vi "Set Last Temperatures.vi"(6 "Read Channel Ident":string, 8 "error in":errorcluster, 9 "Temperatures":dbl[][](array[numeric]), 10 "Channel Idents":string[](array[string]), 11 "Thermometer DAQmx RTD Cont CFG in":refnum<class "Thermometer DAQmx RTD Cont CFG.lvclass">) -> (0 "error out":errorcluster, 1 "Temperature":dbl, 3 "Thermometer DAQmx RTD Cont CFG out":refnum<class "Thermometer DAQmx RTD Cont CFG.lvclass">)   [LabVIEW 2023, in "Thermometer DAQmx RTD Cont CFG.lvclass"]
uses:
  Thermometer DAQmx RTD Cont CFG.lvclass
  Thermometer DAQmx RTD Cont CFG.lvclass/Thermometer DAQmx RTD Cont CFG.ctl
  <vilib>/Analysis/baseanly.llb/Mean (DBL).vi
  <vilib>/Analysis/NI_AALBase.lvlib
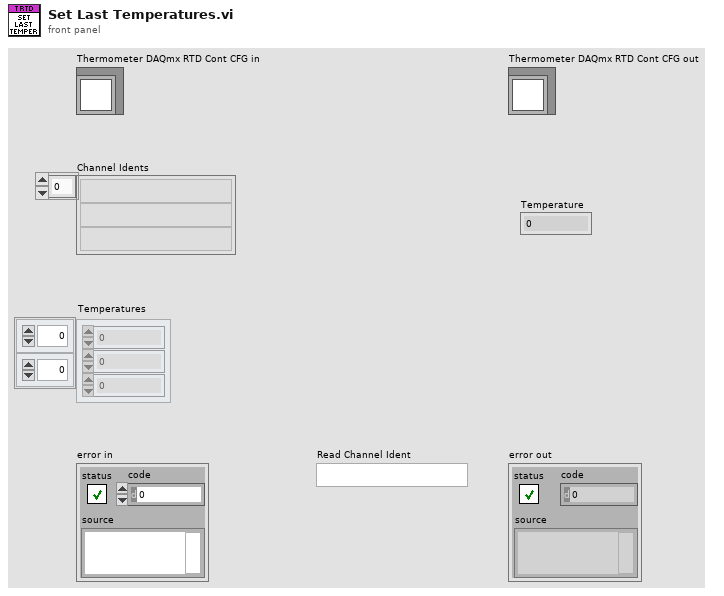
[diagram p1: front panel]
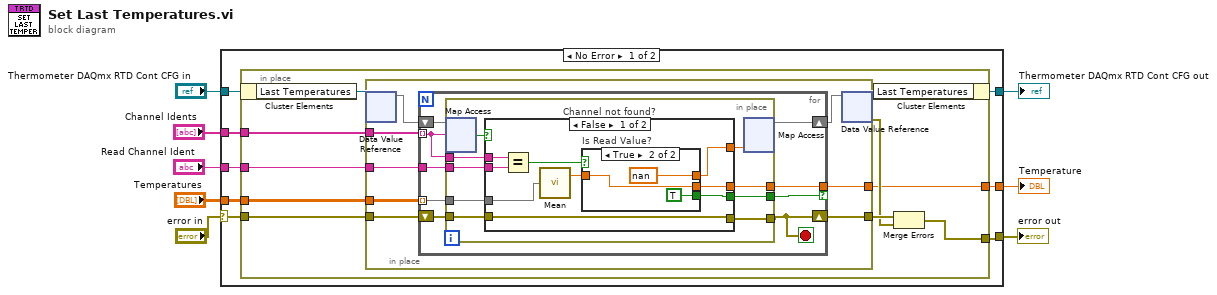
[diagram p0: block diagram]
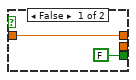
[diagram p2: hidden frame]
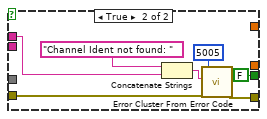
[diagram p3: hidden frame]
diagram:
  n1 = case shown="No Error" "error in" {
    selector: "error in" -> [w14 w75]
    tunnel: [w13 w75] -> w7
    tunnel: [w12 w74] -> w5
    tunnel: "Thermometer DAQmx RTD Cont CFG in" -> [w16 w74]
    tunnel: "Temperatures" -> [w15 _]
    tunnel: "Channel Idents" -> [w11 _]
    tunnel: "Read Channel Ident" -> [w10 _]
    tunnel: [w9 _] -> w1
    frame No Error {
      n2 = in-place {
        in-place-border: w15 -> [w25]
        in-place-border: w14 -> [w24]
        in-place-border: [w21] -> w13
        in-place-border: w11 -> [w19]
        in-place-border: w10 -> [w18]
        in-place-border: [w17] -> w9
        n3 = in-place-cluster #1(w16) -> ("Last Temperatures"=w26:refnum<data-value>)
        n4 = in-place {
          in-place-border: w25 -> [w33]
          in-place-border: w24 -> [w34]
          in-place-border: [w32] -> w23
          in-place-border: w19 -> [w30]
          in-place-border: w18 -> [w28]
          in-place-border: [w27] -> w17
          n5 = in-place-dvr #2(w26) -> (w31:map{string, dbl})  [unwired: 1 out]
          n6 = for {
            tunnel: w33 -> [w42] mode=indexing
            shift-right: [w35] -> w32
            shift-left: w34 -> [w43]
            tunnel: w30 -> [w40] mode=indexing
            shift-right: [w39] -> w29
            shift-left: w31 -> [w41]
            tunnel: w28 -> [w38]
            tunnel: [w37] -> w27 if=w36
            stop <- w35 stop-if-true
            n7 = in-place {
              in-place-border: w43 -> [w52]
              in-place-border: w42 -> [w51]
              in-place-border: [w50] -> w35
              in-place-border: w40 -> [w48]
              in-place-border: w38 -> [w47]
              in-place-border: [w45] -> w37
              in-place-border: [w44] -> w36
              n8 = in-place-map #3(w41, w40) -> (w49:bool)  [unwired: 1 in, 1 out]
              n9 = case "Channel not found?" shown="False" w49 {
                tunnel: w52 -> [w61 w73]
                tunnel: w51 -> [w55 _]
                tunnel: [w61 w69] -> w50
                tunnel: w48 -> [w59 w68]
                tunnel: w47 -> [w60 _]
                tunnel: [w54 _] -> w46
                tunnel: [w57 _] -> w45
                tunnel: [w53 FALSE] -> w44
                frame False {
                  n10 = Equal?(x=w59, y=w60) -> (x = y?=w58:bool)
                  n11 = call-poly <vilib>:"Mean.vi"("X"=w55) -> ("mean"=w56:dbl)  [unwired: 1 out]
                  n12 = case "Is Read Value?" shown="True" w58 {
                    tunnel: [w63 nan] -> w54
                    tunnel: [_ w65] -> w57
                    tunnel: w56 -> [w63 w65]
                    tunnel: [FALSE TRUE] -> w53
                    frame False {
                    }
                    frame True {
                    }
                  }
                }
                frame True {
                  n13 = Concatenate Strings("Channel Ident not found: " ("error message (\"\")"), w68) -> (w71:string)
                  n14 = call <vilib>:"Error Cluster From Error Code.vi"("error in (no error)"=w73, "error message (\"\")"=w71, "error code (0)"=5005) -> ("error out"=w69:errorcluster)  [unwired: 6 in]
                }
              }
              n15 = in-place-map #3(w46) -> (w39:map{string, dbl})  [unwired: 1 in, 2 out]
            }
          }
          n16 = in-place-dvr #2(w29) -> (w22:refnum<data-value>, w20:errorcluster)
        }
        n17 = in-place-cluster #1("Last Temperatures"=w22) -> (w12:refnum<class "Thermometer DAQmx RTD Cont CFG.lvclass">)
        n18 = Merge Errors(w23, w20) -> (w21:errorcluster)
      }
    }
    frame Error {
    }
  }
  "error out" <- w7
  "Thermometer DAQmx RTD Cont CFG out" <- w5
  "Temperature" <- w1
